vi "Set Output Lines.vi"(8 "Error In":errorcluster, 9 "Start Index":i32, 10 "DO Lines":bool[](array[boolean]), 11 "BNT_ULx-MCSV in":refnum<class "BNT_ULx-MCSV.lvclass">) -> (0 "Error Out":errorcluster, 3 "BNT_ULx-MCSV out":refnum<class "BNT_ULx-MCSV.lvclass">)   [LabVIEW 2021, in "BNT_ULx.lvlib" / "BNT_ULx-MCSV.lvclass"]
doc: "Write line values to DAQmx device and publish.\n\nTimeout is set to constant 1s."
uses:
  BNT_ULx-MCSV.lvclass
  BNT_ULx-MCSV.lvclass/BNT_ULx-MCSV.ctl
  <vilib>/ULx/Write.llb/ULx Write (Digital 1D Bool NChan 1Samp 1Line).vi
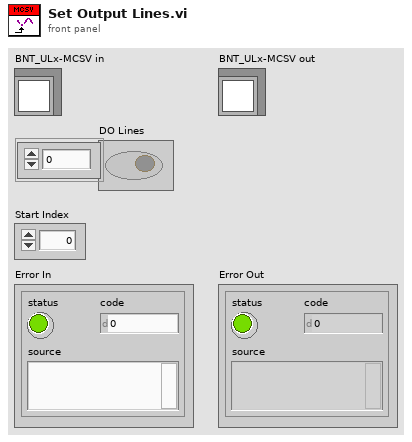
[diagram p1: front panel]
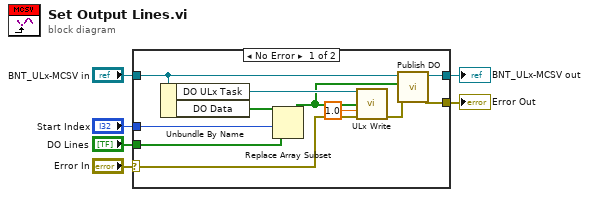
[diagram p0: block diagram]
diagram:
  n1 = case shown="No Error" "Error In" {
    selector: "Error In" -> [w11 w19]
    tunnel: [w12 w19] -> w5
    tunnel: [w14 w18] -> w3
    tunnel: "BNT_ULx-MCSV in" -> [w13 w18]
    tunnel: "DO Lines" -> [w16 _]
    tunnel: "Start Index" -> [w15 _]
    frame No Error {
      n2 = Unbundle By Name(w13) -> ("DO ULx Task"=w9:refnum<k24>, "DO Data"=w17:bool[])
      n3 = Replace Array Subset(array=w17, new element=w16, index=w15) -> (w7:bool[])
      n4 = call-poly <vilib>:"ULx Write.vi"("task in"=w9, "data"=w7, "timeout"=1.0, "error in"=w11) -> ("error out"=w10:errorcluster)  [unwired: 9 in, 2 out]
      n5 = call "Publish DO.vi"("error in"=w10, "DO Data"=w7, "BNT_ULx-MCSV in"=w13) -> ("error out"=w12:errorcluster, "BNT_ULx-MCSV out"=w14:refnum<class "BNT_ULx-MCSV.lvclass">)  [unwired: 7 in]
    }
    frame Error {
    }
  }
  "Error Out" <- w5
  "BNT_ULx-MCSV out" <- w3
